vi "rs232_build_visa_resource_name.vi"(7 "test mode":bool, 9 "19052 COM settings":T1, 11 "19572 COM settings":T1) -> (1 "VISA Resource name 2":refnum<visa-resource-name>, 3 "VISA Resource name 1":refnum<visa-resource-name>)   [LabVIEW 2015]
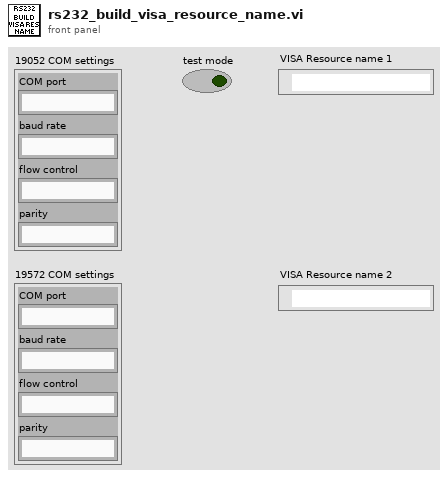
[diagram p1: front panel]
types:
  T1 = cluster{"COM port":string, "baud rate":string, "flow control":string, "parity":string}
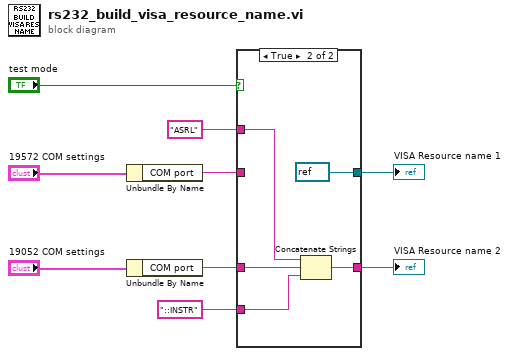
[diagram p0: block diagram]
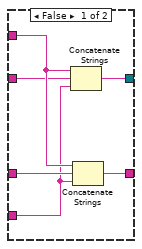
[diagram p2: hidden frame]
diagram:
  n1 = Unbundle By Name("19572 COM settings") -> ("COM port"=w5:string)
  n2 = Unbundle By Name("19052 COM settings") -> ("COM port"=w4:string)
  n3 = case shown="True" "test mode" {
    tunnel: w5 -> [w10 _]
    tunnel: w4 -> [w15 w20]
    tunnel: [w14 refnum<visa-resource-name> refnum ("VISA res out 2")] -> w7
    tunnel: [w13 w18] -> w3
    tunnel: "ASRL" -> [w12 w17]
    tunnel: "::INSTR" -> [w11 w16]
    frame False {
      n4 = Concatenate Strings(w12, w10, w11) -> (w14:string)
      n5 = Concatenate Strings(w12, w15, w11) -> (w13:string)
    }
    frame True {
      n6 = Concatenate Strings(w17, w20, w16) -> (w18:string)
    }
  }
  "VISA Resource name 2" <- w3
  "VISA Resource name 1" <- w7
